vi "1.vi"() -> ()   [LabVIEW 2023]
uses:
  TYPEDEF_COFFEE.ctl
  Control Timer.ctl
panel:
  out "error out":errorcluster
  in  "STOP":bool
  in  "WHITE COFFEE":bool
  in  "CAPUCCINO":bool
  in  "ESPRESSO LONG":bool
  in  "ESPRESSO SHORT":bool
  out "RELEASE ALL":bool
  out "MIXING":bool
  out "BOILING MILK":bool
  out "ADDING MILK":bool
  out "BOILING":bool
  out "ADDING COFFEE":bool
  out "ADDING WATER":bool
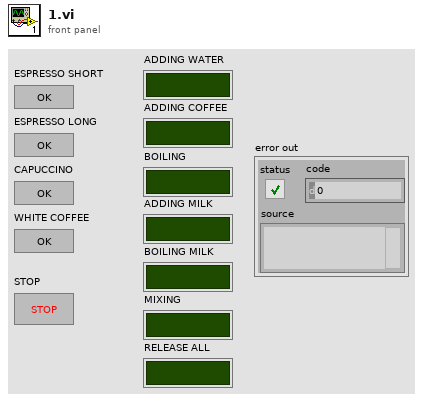
[diagram p1: front panel]
types:
  T1 = typedef "TYPEDEF_COFFEE.ctl" = enum16{"INIT", "WAIT", "SHUTDOWN", "ADDING WATER", "ADDING COFFEE", "BOILING", "ADDING MILK", "BOILING MILK", "MIXING", "RELEASE ALL"}
  T2 = typedef "Control Timer.ctl" = enum16{"Timecheck", "Reset"}
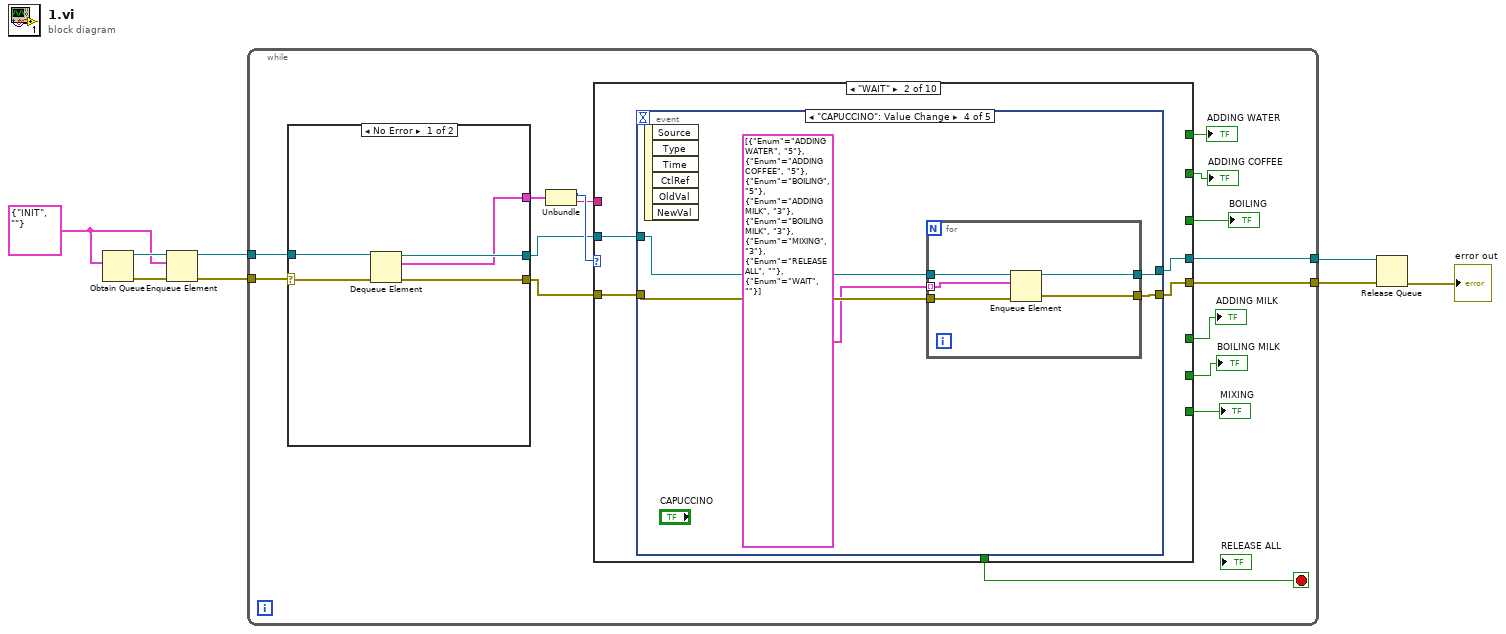
[diagram p0: block diagram]
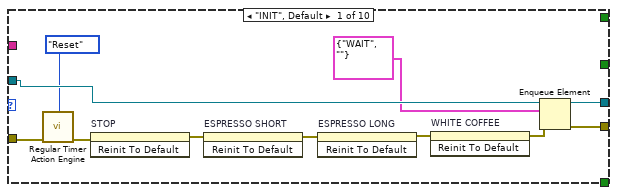
[diagram p2: hidden frame]
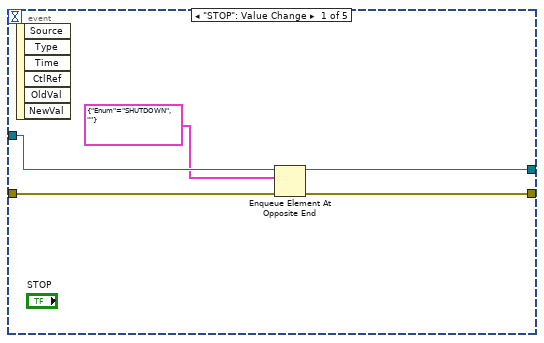
[diagram p3: hidden frame]
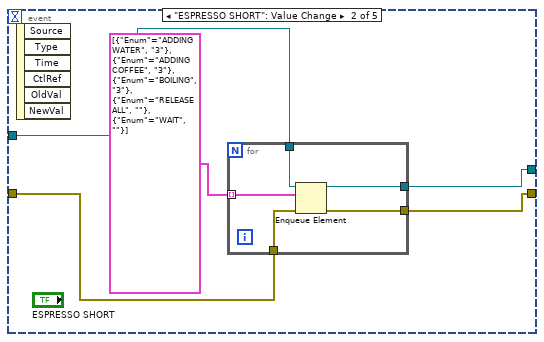
[diagram p4: hidden frame]
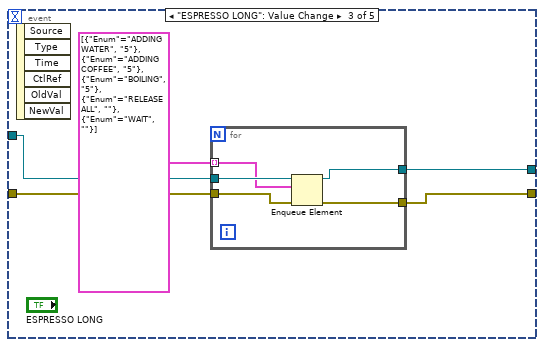
[diagram p5: hidden frame]
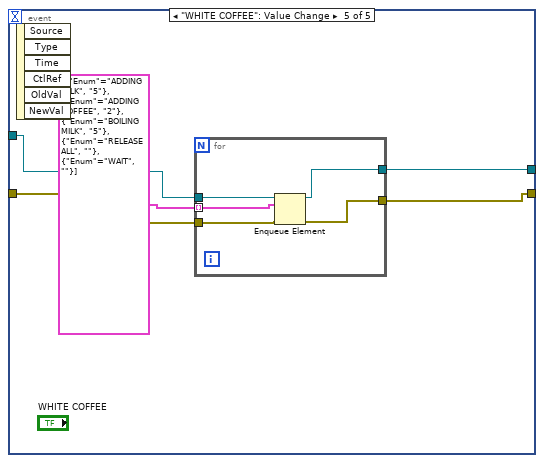
[diagram p6: hidden frame]
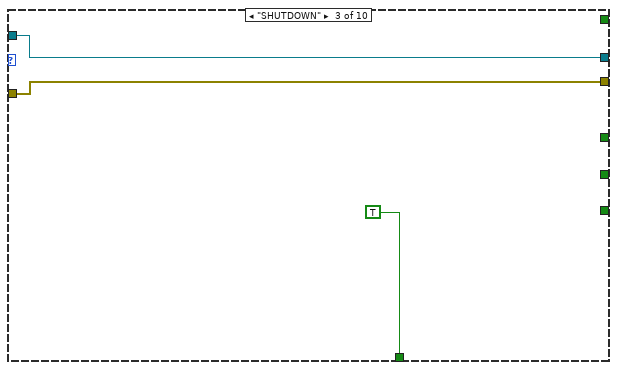
[diagram p7: hidden frame]
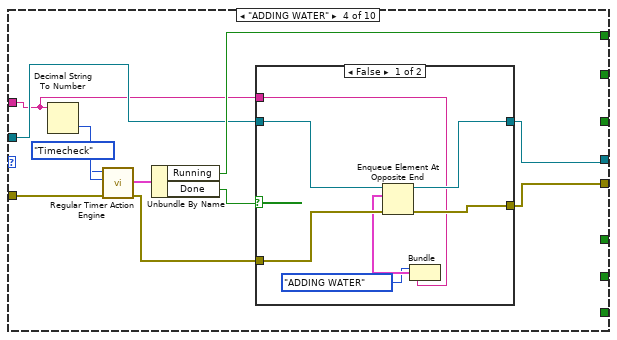
[diagram p8: hidden frame]
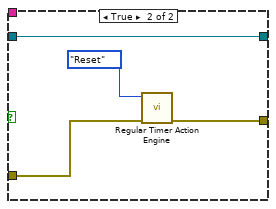
[diagram p9: hidden frame]
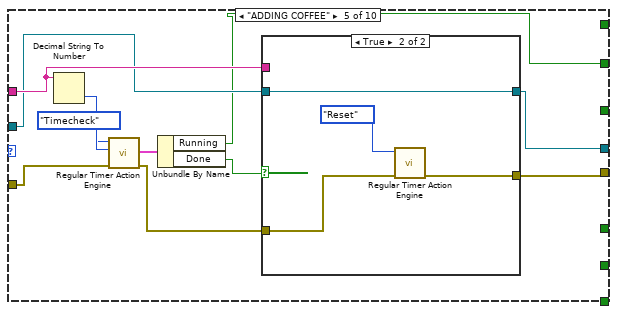
[diagram p10: hidden frame]
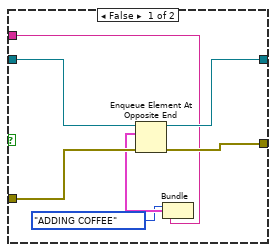
[diagram p11: hidden frame]
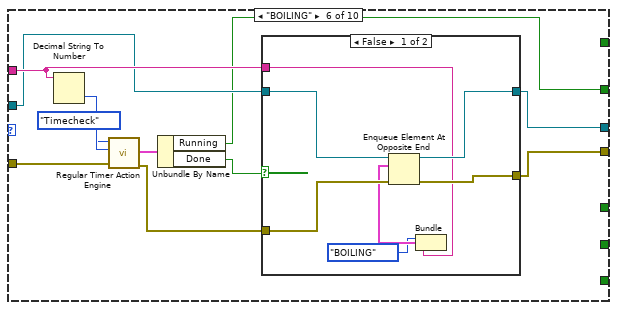
[diagram p12: hidden frame]
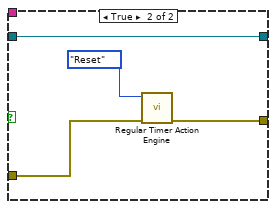
[diagram p13: hidden frame]
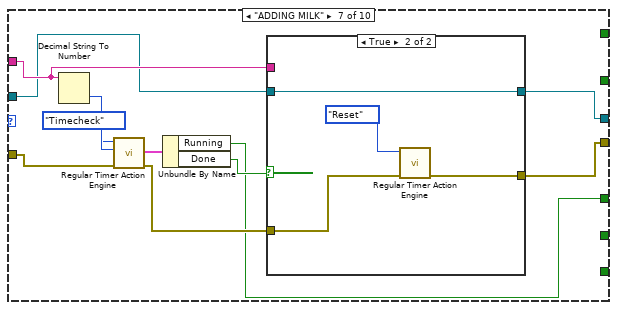
[diagram p14: hidden frame]
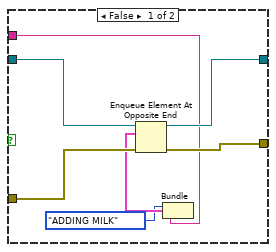
[diagram p15: hidden frame]
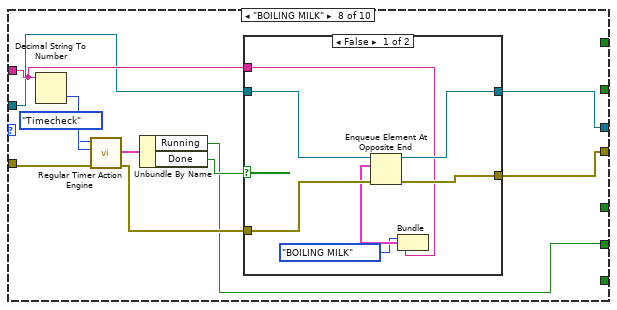
[diagram p16: hidden frame]
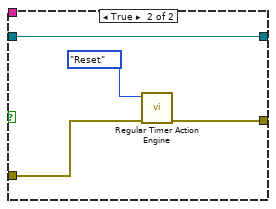
[diagram p17: hidden frame]
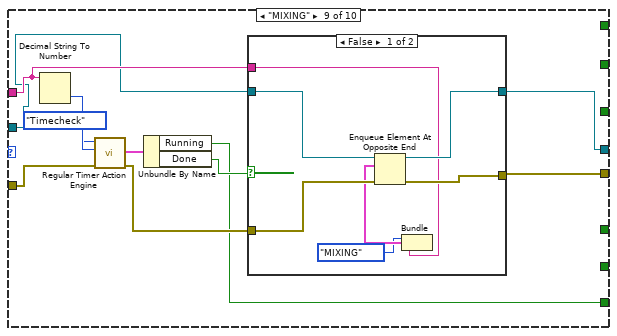
[diagram p18: hidden frame]
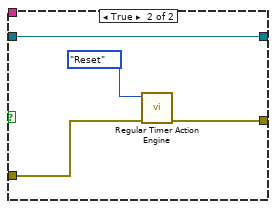
[diagram p19: hidden frame]
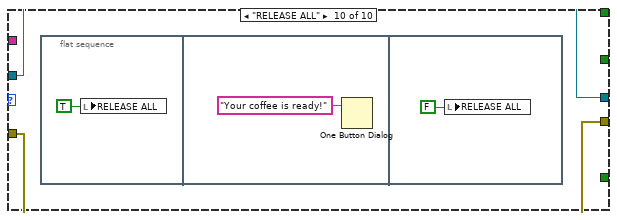
[diagram p20: hidden frame]
diagram:
  w6 = cluster{"Enum":T1, string} {"Enum"=enum."INIT", ""}
  n1 = Obtain Queue(element data type=w6) -> (queue out=w7:refnum<queue>, error out=w8:errorcluster)  [unwired: 4 in, 1 out]
  n2 = Enqueue Element(queue=w7, element=w6, error in (no error)=w8) -> (queue out=w4:refnum<queue>, error out=w5:errorcluster)  [unwired: 1 in, 1 out]
  n3 = while {
    tunnel: w5 -> [w24]
    tunnel: w4 -> [w23]
    tunnel: [w17] -> w2
    tunnel: [w16] -> w3
    stop <- w18 stop-if-true
    n4 = case shown="No Error" w24 {
      selector: w24 -> [w229 w234]
      tunnel: w23 -> [w228 w233]
      tunnel: [w227 w231] -> w19
      tunnel: [w226 w232] -> w20
      tunnel: [w225 w230] -> w22
      frame No Error {
        n5 = Dequeue Element(queue=w228, error in (no error)=w229) -> (queue out=w226:refnum<queue>, element=w225:cluster{"Enum":T1, string}, error out=w227:errorcluster)  [unwired: 1 in, 1 out]
      }
      frame Error {
        w230 = cluster{"Enum":T1, string} {"Enum"=enum."SHUTDOWN", ""}
        n6 = Enqueue Element At Opposite End(queue=w233, element=w230, error in (no error)=w234) -> (queue out=w232:refnum<queue>, error out=w231:errorcluster)  [unwired: 1 in, 1 out]
      }
    }
    n7 = Unbundle(w22) -> ("Enum"=w21:T1, w15:string)
    n8 = case shown="\"WAIT\"" w21 {
      tunnel: w20 -> [w35 w38 w85 w90 w114 w136 w157 w179 w201 w221]
      tunnel: w19 -> [w26 w39 w86 w98 w113 w135 w159 w181 w203 w220]
      tunnel: [w33 w36 w85 w89 w111 w133 w156 w177 w200 w221] -> w17
      tunnel: [w32 w37 w86 w91 w112 w134 w155 w176 w199 w220] -> w16
      tunnel: [_ _ TRUE _ _ _ _ _ _ _] -> w18
      tunnel: w15 -> [_ _ _ w88 w115 w137 w158 w180 w202 _]
      tunnel: [_ _ _ w94 _ _ _ _ _ _] -> w14
      tunnel: [_ _ _ _ w110 _ _ _ _ _] -> w13
      tunnel: [_ _ _ _ _ w132 _ _ _ _] -> w12
      tunnel: [_ _ _ _ _ _ w154 _ _ _] -> w11
      tunnel: [_ _ _ _ _ _ _ w178 _ _] -> w10
      tunnel: [_ _ _ _ _ _ _ _ w198 _] -> w9
      frame "INIT", Default {
        n9 = call "Regular Timer Action Engine.vi"("Enum"=Control_Timer."Reset", "error in"=w26) -> ("error out"=w27:errorcluster)  [unwired: 7 in, 1 out]
        n10 = invoke on="STOP" class="Bool" method="Reinit To Default"(error in=w27) -> (error out=w31:errorcluster)  [unwired: 2 in, 2 out]
        n11 = invoke on="ESPRESSO SHORT" class="Bool" method="Reinit To Default"(error in=w31) -> (error out=w30:errorcluster)  [unwired: 2 in, 2 out]
        n12 = invoke on="ESPRESSO LONG" class="Bool" method="Reinit To Default"(error in=w30) -> (error out=w29:errorcluster)  [unwired: 2 in, 2 out]
        n13 = invoke on="WHITE COFFEE" class="Bool" method="Reinit To Default"(error in=w29) -> (error out=w28:errorcluster)  [unwired: 2 in, 2 out]
        n14 = Enqueue Element(queue=w35, element=cluster{"Enum":T1, string} {"Enum"=enum."WAIT", ""}, error in (no error)=w28) -> (queue out=w33:refnum<queue>, error out=w32:errorcluster)  [unwired: 1 in, 1 out]
      }
      frame "WAIT" {
        n15 = event shown="[3] \"CAPUCCINO\": Value Change" {
          selector: _ -> [_ _ _ _ _]
          dyn-events: _ -> [_ _ _ _ _]
          timeout: _ -> [_ _ _ _ _]
          tunnel: w39 -> [w44 w48 w58 w69 w77]
          tunnel: w38 -> [w43 w49 w59 w68 w76]
          tunnel: [w41 w46 w57 w67 w79] -> w36
          tunnel: [w40 w45 w56 w66 w78] -> w37
          event "STOP": Value Change {
            n16 = event-data() -> ()  [unwired: 1 in, 6 out]
            n17 = Enqueue Element At Opposite End(queue=w43, element=cluster{"Enum":T1, string} {"Enum"=enum."SHUTDOWN", ""}, error in (no error)=w44) -> (queue out=w41:refnum<queue>, error out=w40:errorcluster)  [unwired: 1 in, 1 out]
          }
          event "ESPRESSO SHORT": Value Change {
            n18 = event-data() -> ()  [unwired: 1 in, 6 out]
            n19 = for {
              tunnel: w49 -> [w54]
              tunnel: w48 -> [w53]
              tunnel: cluster{"Enum":T1, string}[] [{"Enum"=enum."ADDING WATER", "3"}, {"Enum"=enum."ADDING COFFEE", "3"}, {"Enum"=enum."BOILING", "3"}, {"Enum"=enum."RELEASE ALL", ""}, {"Enum"=enum."WAIT", ""}] -> [w52] mode=indexing
              tunnel: [w51] -> w46
              tunnel: [w50] -> w45
              n20 = Enqueue Element(queue=w54, element=w52, error in (no error)=w53) -> (queue out=w51:refnum<queue>, error out=w50:errorcluster)  [unwired: 1 in, 1 out]
            }
          }
          event "ESPRESSO LONG": Value Change {
            n21 = event-data() -> ()  [unwired: 1 in, 6 out]
            n22 = for {
              tunnel: w59 -> [w64]
              tunnel: w58 -> [w63]
              tunnel: [w62] -> w57
              tunnel: [w61] -> w56
              tunnel: cluster{"Enum":T1, string}[] [{"Enum"=enum."ADDING WATER", "5"}, {"Enum"=enum."ADDING COFFEE", "5"}, {"Enum"=enum."BOILING", "5"}, {"Enum"=enum."RELEASE ALL", ""}, {"Enum"=enum."WAIT", ""}] -> [w60] mode=indexing
              n23 = Enqueue Element(queue=w64, element=w60, error in (no error)=w63) -> (queue out=w62:refnum<queue>, error out=w61:errorcluster)  [unwired: 1 in, 1 out]
            }
          }
          event "CAPUCCINO": Value Change {
            n24 = event-data() -> ()  [unwired: 1 in, 6 out]
            n25 = for {
              tunnel: w69 -> [w74]
              tunnel: w68 -> [w73]
              tunnel: [w72] -> w67
              tunnel: [w71] -> w66
              tunnel: cluster{"Enum":T1, string}[] [{"Enum"=enum."ADDING WATER", "5"}, {"Enum"=enum."ADDING COFFEE", "5"}, {"Enum"=enum."BOILING", "5"}, {"Enum"=enum."ADDING MILK", "3"}, {"Enum"=enum."BOILING MILK", "3"}, {"Enum"=enum."MIXING", "3"}, {"Enum"=enum."RELEASE ALL", ""}, {"Enum"=enum."WAIT", ""}] -> [w70] mode=indexing
              n26 = Enqueue Element(queue=w73, element=w70, error in (no error)=w74) -> (queue out=w72:refnum<queue>, error out=w71:errorcluster)  [unwired: 1 in, 1 out]
            }
          }
          event "WHITE COFFEE": Value Change {
            n27 = event-data() -> ()  [unwired: 1 in, 6 out]
            n28 = for {
              tunnel: [w84] -> w79
              tunnel: [w83] -> w78
              tunnel: w77 -> [w82]
              tunnel: w76 -> [w81]
              tunnel: cluster{"Enum":T1, string}[] [{"Enum"=enum."ADDING MILK", "5"}, {"Enum"=enum."ADDING COFFEE", "2"}, {"Enum"=enum."BOILING MILK", "5"}, {"Enum"=enum."RELEASE ALL", ""}, {"Enum"=enum."WAIT", ""}] -> [w80] mode=indexing
              n29 = Enqueue Element(queue=w81, element=w80, error in (no error)=w82) -> (queue out=w84:refnum<queue>, error out=w83:errorcluster)  [unwired: 1 in, 1 out]
            }
          }
        }
      }
      frame "SHUTDOWN" {
      }
      frame "ADDING WATER" {
        n30 = Decimal String To Number(string=w88) -> (number=w97:i32)  [unwired: 2 in, 1 out]
        n31 = call "Regular Timer Action Engine.vi"("Enum"=Control_Timer."Timecheck", "Time Target"=w97, "error in"=w98) -> ("Status"=w95:cluster{"Running":bool, "Done":bool}, "error out"=w92:errorcluster)  [unwired: 6 in]
        n32 = Unbundle By Name(w95) -> ("Running"=w94:bool, "Done"=w93:bool)
        n33 = case shown="False" w93 {
          tunnel: w92 -> [w105 w109]
          tunnel: [w102 w107] -> w91
          tunnel: w90 -> [w104 w106]
          tunnel: [w103 w106] -> w89
          tunnel: w88 -> [w99 _]
          frame False {
            n34 = Bundle("Enum"=TYPEDEF_COFFEE."ADDING WATER", w99) -> (w101:cluster{"Enum":T1, string})  [unwired: 1 in]
            n35 = Enqueue Element At Opposite End(queue=w104, element=w101, error in (no error)=w105) -> (queue out=w103:refnum<queue>, error out=w102:errorcluster)  [unwired: 1 in, 1 out]
          }
          frame True {
            n36 = call "Regular Timer Action Engine.vi"("Enum"=Control_Timer."Reset", "error in"=w109) -> ("error out"=w107:errorcluster)  [unwired: 7 in, 1 out]
          }
        }
      }
      frame "ADDING COFFEE" {
        n37 = Decimal String To Number(string=w115) -> (number=w120:i32)  [unwired: 2 in, 1 out]
        n38 = call "Regular Timer Action Engine.vi"("Enum"=Control_Timer."Timecheck", "Time Target"=w120, "error in"=w113) -> ("Status"=w118:cluster{"Running":bool, "Done":bool}, "error out"=w116:errorcluster)  [unwired: 6 in]
        n39 = Unbundle By Name(w118) -> ("Running"=w110:bool, "Done"=w117:bool)
        n40 = case shown="True" w117 {
          tunnel: w116 -> [w127 w131]
          tunnel: [w124 w129] -> w112
          tunnel: w114 -> [w126 w128]
          tunnel: [w125 w128] -> w111
          tunnel: w115 -> [w121 _]
          frame False {
            n41 = Bundle("Enum"=TYPEDEF_COFFEE."ADDING COFFEE", w121) -> (w123:cluster{"Enum":T1, string})  [unwired: 1 in]
            n42 = Enqueue Element At Opposite End(queue=w126, element=w123, error in (no error)=w127) -> (queue out=w125:refnum<queue>, error out=w124:errorcluster)  [unwired: 1 in, 1 out]
          }
          frame True {
            n43 = call "Regular Timer Action Engine.vi"("Enum"=Control_Timer."Reset", "error in"=w131) -> ("error out"=w129:errorcluster)  [unwired: 7 in, 1 out]
          }
        }
      }
      frame "BOILING" {
        n44 = Decimal String To Number(string=w137) -> (number=w142:i32)  [unwired: 2 in, 1 out]
        n45 = call "Regular Timer Action Engine.vi"("Enum"=Control_Timer."Timecheck", "Time Target"=w142, "error in"=w135) -> ("Status"=w140:cluster{"Running":bool, "Done":bool}, "error out"=w138:errorcluster)  [unwired: 6 in]
        n46 = Unbundle By Name(w140) -> ("Running"=w132:bool, "Done"=w139:bool)
        n47 = case shown="False" w139 {
          tunnel: w138 -> [w149 w153]
          tunnel: [w146 w151] -> w134
          tunnel: w136 -> [w148 w150]
          tunnel: [w147 w150] -> w133
          tunnel: w137 -> [w143 _]
          frame False {
            n48 = Bundle("Enum"=TYPEDEF_COFFEE."BOILING", w143) -> (w145:cluster{"Enum":T1, string})  [unwired: 1 in]
            n49 = Enqueue Element At Opposite End(queue=w148, element=w145, error in (no error)=w149) -> (queue out=w147:refnum<queue>, error out=w146:errorcluster)  [unwired: 1 in, 1 out]
          }
          frame True {
            n50 = call "Regular Timer Action Engine.vi"("Enum"=Control_Timer."Reset", "error in"=w153) -> ("error out"=w151:errorcluster)  [unwired: 7 in, 1 out]
          }
        }
      }
      frame "ADDING MILK" {
        n51 = Decimal String To Number(string=w158) -> (number=w164:i32)  [unwired: 2 in, 1 out]
        n52 = call "Regular Timer Action Engine.vi"("Enum"=Control_Timer."Timecheck", "Time Target"=w164, "error in"=w159) -> ("Status"=w162:cluster{"Running":bool, "Done":bool}, "error out"=w160:errorcluster)  [unwired: 6 in]
        n53 = Unbundle By Name(w162) -> ("Running"=w154:bool, "Done"=w161:bool)
        n54 = case shown="True" w161 {
          tunnel: w160 -> [w171 w175]
          tunnel: [w168 w173] -> w155
          tunnel: w157 -> [w170 w172]
          tunnel: [w169 w172] -> w156
          tunnel: w158 -> [w165 _]
          frame False {
            n55 = Bundle("Enum"=TYPEDEF_COFFEE."ADDING MILK", w165) -> (w167:cluster{"Enum":T1, string})  [unwired: 1 in]
            n56 = Enqueue Element At Opposite End(queue=w170, element=w167, error in (no error)=w171) -> (queue out=w169:refnum<queue>, error out=w168:errorcluster)  [unwired: 1 in, 1 out]
          }
          frame True {
            n57 = call "Regular Timer Action Engine.vi"("Enum"=Control_Timer."Reset", "error in"=w175) -> ("error out"=w173:errorcluster)  [unwired: 7 in, 1 out]
          }
        }
      }
      frame "BOILING MILK" {
        n58 = Decimal String To Number(string=w180) -> (number=w186:i32)  [unwired: 2 in, 1 out]
        n59 = call "Regular Timer Action Engine.vi"("Enum"=Control_Timer."Timecheck", "Time Target"=w186, "error in"=w181) -> ("Status"=w184:cluster{"Running":bool, "Done":bool}, "error out"=w182:errorcluster)  [unwired: 6 in]
        n60 = Unbundle By Name(w184) -> ("Running"=w178:bool, "Done"=w183:bool)
        n61 = case shown="False" w183 {
          tunnel: w182 -> [w193 w197]
          tunnel: [w190 w195] -> w176
          tunnel: w179 -> [w192 w194]
          tunnel: [w191 w194] -> w177
          tunnel: w180 -> [w187 _]
          frame False {
            n62 = Bundle("Enum"=TYPEDEF_COFFEE."BOILING MILK", w187) -> (w189:cluster{"Enum":T1, string})  [unwired: 1 in]
            n63 = Enqueue Element At Opposite End(queue=w192, element=w189, error in (no error)=w193) -> (queue out=w191:refnum<queue>, error out=w190:errorcluster)  [unwired: 1 in, 1 out]
          }
          frame True {
            n64 = call "Regular Timer Action Engine.vi"("Enum"=Control_Timer."Reset", "error in"=w197) -> ("error out"=w195:errorcluster)  [unwired: 7 in, 1 out]
          }
        }
      }
      frame "MIXING" {
        n65 = Decimal String To Number(string=w202) -> (number=w208:i32)  [unwired: 2 in, 1 out]
        n66 = call "Regular Timer Action Engine.vi"("Enum"=Control_Timer."Timecheck", "Time Target"=w208, "error in"=w203) -> ("Status"=w206:cluster{"Running":bool, "Done":bool}, "error out"=w204:errorcluster)  [unwired: 6 in]
        n67 = Unbundle By Name(w206) -> ("Running"=w198:bool, "Done"=w205:bool)
        n68 = case shown="False" w205 {
          tunnel: w204 -> [w215 w219]
          tunnel: [w212 w217] -> w199
          tunnel: w201 -> [w214 w216]
          tunnel: [w213 w216] -> w200
          tunnel: w202 -> [w209 _]
          frame False {
            n69 = Bundle("Enum"=TYPEDEF_COFFEE."MIXING", w209) -> (w211:cluster{"Enum":T1, string})  [unwired: 1 in]
            n70 = Enqueue Element At Opposite End(queue=w214, element=w211, error in (no error)=w215) -> (queue out=w213:refnum<queue>, error out=w212:errorcluster)  [unwired: 1 in, 1 out]
          }
          frame True {
            n71 = call "Regular Timer Action Engine.vi"("Enum"=Control_Timer."Reset", "error in"=w219) -> ("error out"=w217:errorcluster)  [unwired: 7 in, 1 out]
          }
        }
      }
      frame "RELEASE ALL" {
        n72 = flat-sequence {
          frame #0 {
            n73 = local write "RELEASE ALL"(TRUE ("RELEASE ALL")) -> ()
          }
          frame #1 {
            n74 = One Button Dialog(message="Your coffee is ready!") -> ()  [unwired: 1 in, 1 out]
          }
          frame #2 {
            n75 = local write "RELEASE ALL"(FALSE ("RELEASE ALL")) -> ()
          }
        }
      }
    }
    "ADDING WATER" <- w14
    "ADDING COFFEE" <- w13
    "BOILING" <- w12
    "ADDING MILK" <- w11
    "BOILING MILK" <- w10
    "MIXING" <- w9
  }
  n76 = Release Queue(queue=w2, error in (no error)=w3) -> (error out=→"error out":errorcluster)  [unwired: 1 in, 2 out]
